vi "RT_Aerodynamic_Force_in_DLR_Navigation_Reference_System (SubVI).vi"(0 "Data":dbl[][](array[numeric]), 1 "AoA_pitch (rad)":dbl, 2 "AoA_yaw (rad)":dbl, 5 "i":i32, 9 "DCM":dbl[][](array[numeric]), 11 "Sref [m^2]":dbl, 13 "Pdin":dbl) -> (4 "FA":dbl[](array[numeric]), 15 "FA_b":dbl[](array[numeric]))   [LabVIEW 2011]
uses:
  <vilib>/Analysis/coordinate.llb/Euler Rotation Order.ctl
  <vilib>/Analysis/Matrix/Numeric/Conversions/Array To Matrix - RA2.vi
  <vilib>/Analysis/Matrix/Numeric/Conversions/Array To Matrix - RA.vi
  <vilib>/Analysis/baseanly.llb/Real A x B.vi
  <vilib>/Analysis/Matrix/Numeric/Conversions/Matrix To Array - RM.vi
  <vilib>/Analysis/NI_AALPro.lvlib
  <vilib>/Analysis/Matrix/NI_Matrix.lvlib
  <vilib>/Analysis/NI_AALBase.lvlib
panel:
  out "FAl":dbl[](array[numeric])
  out "FAy":dbl[](array[numeric])
  out "FAp":dbl[](array[numeric])
  out "FA_long":dbl
  out "FA_yaw":dbl
  out "FA_pitch":dbl
  out "Sref - Area de referencia":dbl=1.72 format="%#_13g"
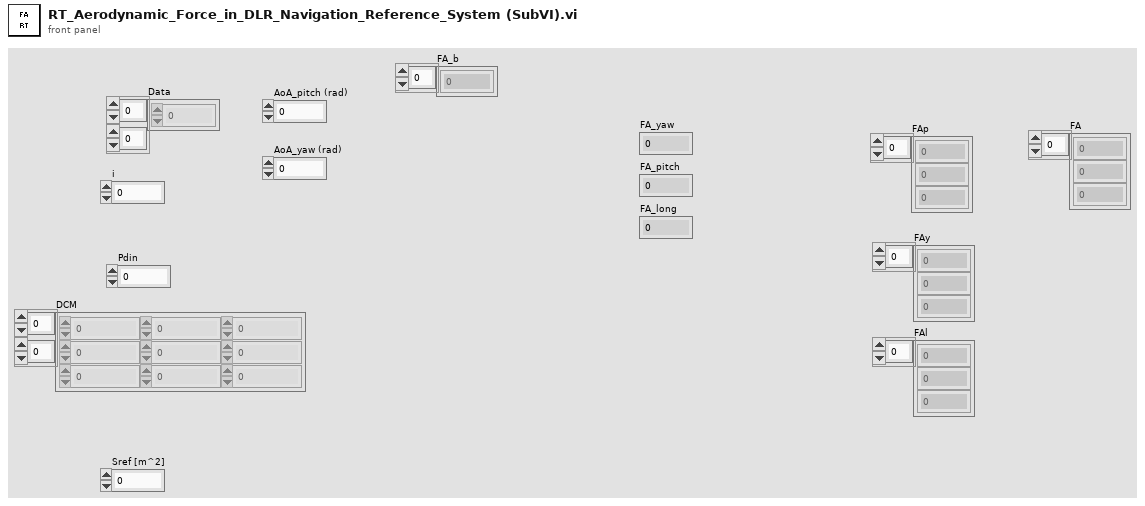
[diagram p1: front panel]
types:
  T1 = typedef "NI_AALPro.lvlib/Euler Rotation Order.ctl" = u16
  T2 = typedef "NI_Matrix.lvlib/RealMatrix.ctl" = dbl[][]
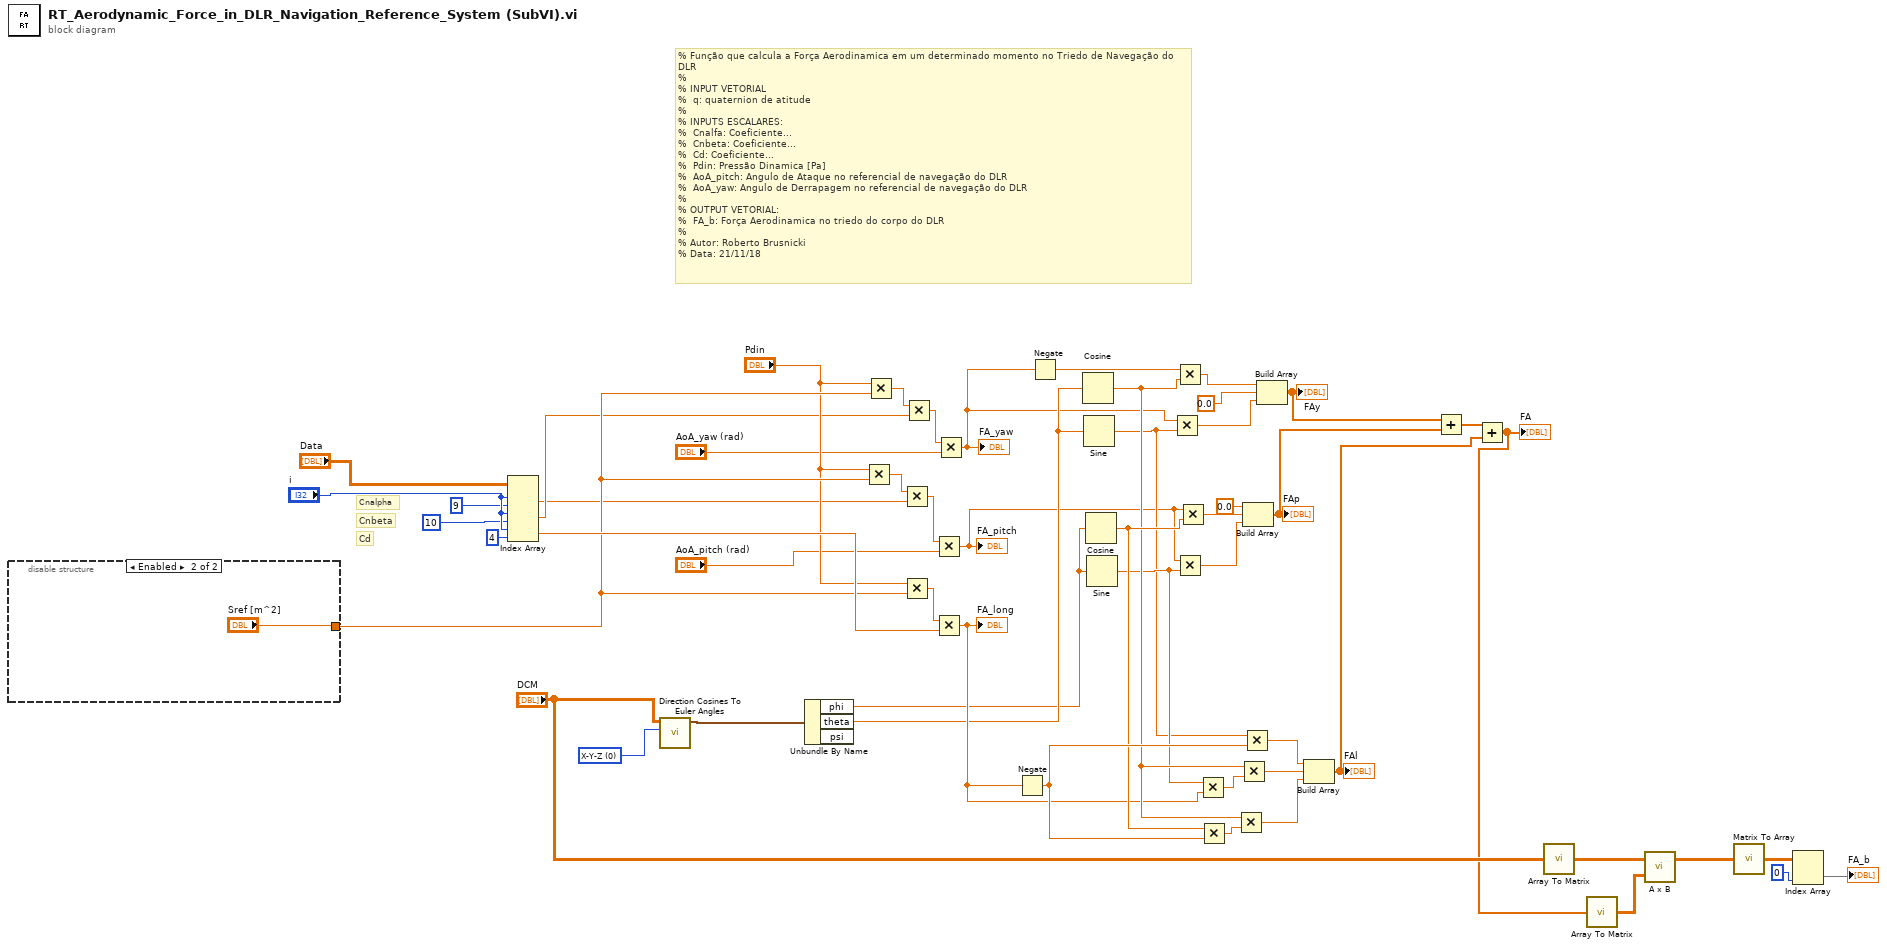
[diagram p0: block diagram]
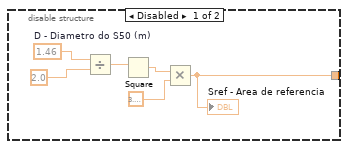
[diagram p2: hidden frame]
diagram:
  w14 = T1 0 items=["X-Y-Z", "X-Z-Y", "Y-X-Z", "Y-Z-X", "Z-X-Y", "Z-Y-X", "X-Y-X", "X-Z-X", "Y-X-Y", "Y-Z-Y", "Z-X-Z", "Z-Y-Z"] ("rotation order")
  # "% Função que calcula a Força Aerodinamica em um determinado momento no Triedo de Navegação do DLR\n%\n% INPUT VETORIAL\n%  q: quaternion de atitude\n%\n% INPUTS ESCALARES:\n%  Cnalfa: Coeficiente...\n%  Cnbeta: Coeficiente...\n%  Cd: Coeficiente...\n%  Pdin: Pressão Dinamica [Pa]\n%  AoA_pitch: Angulo de Ataque no referencial de navegação do DLR\n%  AoA_yaw: Angulo de Derrapagem no referencial de navegação do DLR\n%\n% OUTPUT VETORIAL:\n%  FA_b: Força Aerodinamica no triedo do corpo do DLR\n%\n% Autor: Roberto Brusnicki\n% Data: 21/11/18"
  # "Cd"
  # "Cnbeta"
  # "Cnalpha"
  n1 = disable-structure shown="Enabled" {
    disable-tunnel: [w59 "Sref [m^2]"] -> w25
    frame Disabled {
      w54 = 1.46  # D - Diametro do S50 (m)
      n2 = Divide(x=w54, y=2.0) -> (x/y=w57:dbl)
      n3 = Square(x=w57) -> (x^2=w58:dbl)
      n4 = Multiply(x=w58, y=3.141592653589793) -> (x*y=w59:dbl)
      "Sref - Area de referencia" <- w59
    }
    frame Enabled {
    }
  }
  n5 = Index Array(array="Data", index (row) #1="i", index (col) #1=9 ("disabled index (col)"), index (row) #2="i", index (col) #2=10 ("disabled index (col)"), index (row) #3="i", index (col) #3=4 ("disabled index (col)")) -> (element #1=w15:dbl, element #2=w21:dbl, element #3=w26:dbl)
  n6 = call <vilib>:"Direction Cosines To Euler Angles.vi"("rotation order"=w14, "Direction Cosines"="DCM") -> ("Euler Angles"=w27:cluster{"phi":dbl, "theta":dbl, "psi":dbl})  [unwired: 8 in, 1 out]
  n7 = Unbundle By Name(w27) -> ("phi"=w29:dbl, "theta"=w35:dbl)  [unwired: 1 out]
  n8 = Multiply(x="Pdin", y=w25) -> (x*y=w16:dbl)
  n9 = Multiply(x="Pdin", y=w25) -> (x*y=w20:dbl)
  n10 = Multiply(x=w16, y=w15) -> (x*y=w18:dbl)
  n11 = Multiply(x="Pdin", y=w25) -> (x*y=w23:dbl)
  n12 = Multiply(x=w20, y=w21) -> (x*y=w19:dbl)
  n13 = Multiply(x=w18, y="AoA_pitch (rad)") -> (x*y=w28:dbl)
  "FA_pitch" <- w28
  n14 = Multiply(x=w23, y=w26) -> (x*y=w45:dbl)
  "FA_long" <- w45
  n15 = Multiply(x=w19, y="AoA_yaw (rad)") -> (x*y=w33:dbl)
  "FA_yaw" <- w33
  n16 = Negate(x=w45) -> (-x=w49:dbl)
  n17 = Negate(x=w33) -> (-x=w34:dbl)
  n18 = Cosine(x=w35) -> (cos(x)=w46:dbl)
  n19 = Sine(x=w35) -> (sin(x)=w42:dbl)
  n20 = Cosine(x=w29) -> (cos(x)=w48:dbl)
  n21 = Sine(x=w29) -> (sin(x)=w44:dbl)
  n22 = Multiply(x=w33, y=w42) -> (x*y=w37:dbl)
  n23 = Multiply(x=w34, y=w46) -> (x*y=w36:dbl)
  n24 = Multiply(x=w28, y=w44) -> (x*y=w30:dbl)
  n25 = Multiply(x=w28, y=w48) -> (x*y=w31:dbl)
  n26 = Multiply(x=w44, y=w45) -> (x*y=w43:dbl)
  n27 = Multiply(x=w48, y=w49) -> (x*y=w47:dbl)
  n28 = Multiply(x=w46, y=w47) -> (x*y=w39:dbl)
  n29 = Multiply(x=w46, y=w43) -> (x*y=w40:dbl)
  n30 = Multiply(x=w42, y=w49) -> (x*y=w41:dbl)
  n31 = Build Array(0.0 ("element"), w31, w30) -> (w51:dbl[])
  "FAp" <- w51
  n32 = Build Array(w36, 0.0 ("element"), w37) -> (w50:dbl[])
  "FAy" <- w50
  n33 = Build Array(w41, w40, w39) -> (w53:dbl[])
  "FAl" <- w53
  n34 = Add(x=w50, y=w51) -> (x+y=w52:dbl[])
  n35 = Add(x=w52, y=w53) -> (x+y=w2:dbl[])
  "FA" <- w2
  n36 = call-poly <vilib>:"Array To Matrix.vi"("Real 2D Array"="DCM") -> ("Real Matrix"=w4:T2)
  n37 = call-poly <vilib>:"Array To Matrix.vi"("Real 1D Array"=w2) -> ("Real Matrix (Column Vector)"=w7:T2)
  n38 = call-poly <vilib>:"A x B.vi"("B"=w7, "A"=w4) -> ("A x B"=w6:T2)  [unwired: 1 out]
  n39 = call-poly <vilib>:"Matrix To Array.vi"("Real Matrix"=w6) -> ("Real 2D Array"=w8:dbl[][])
  n40 = Index Array(array=w8, index (col)=0 ("index (row)")) -> (element=→"FA_b":dbl[])  [unwired: 1 in]
